vi "Initialize.vi"(8 "error in (no error)":errorcluster) -> (0 "error out":errorcluster, 3 "DVR":T1)   [LabVIEW 2020, in "DVR-Module.lvlib"]
uses:
  DVR-Module.lvlib
  DVR.ctl
  DataDef.ctl
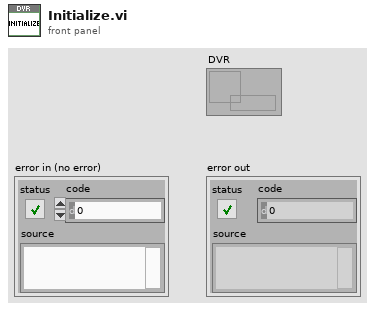
[diagram p1: front panel]
types:
  T1 = typedef "DVR-Module.lvlib/DVR.ctl" = refnum<data-value>
  T2 = typedef "DataDef.ctl" = cluster{"dbl":dbl}
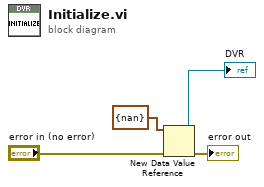
[diagram p0: block diagram]
diagram:
  n1 = New Data Value Reference(data value=T2 {"dbl"=nan} ("ModuleData"), error in="error in (no error)") -> (data value reference=→"DVR":refnum<data-value>, error out=→"error out":errorcluster)
